vi "GetFrontEndStatus.vi"(8 "error in (no error)":errorcluster) -> (0 "error out":errorcluster, 1 "TestSetDef":T2={"General"={"ID"=0, "Model"="", "Dual Port?"=FALSE, "Options"="", "Options"={"E"=FALSE, "K"=FALSE, "H"=FALSE, "W"=FALSE, "F"=FALSE}, "Cal File"=path ""}, "Receiver"={"Fstart, MHz"=0.0, "Fstop MHz"=0.0, "Fstep MHz"=0.0, "IF, MHz"=0.0}, "RX Band"={"Fstart, MHz"=0.0, "Fstop MHz"=0.0}, "TX 1"={"Fstart, MHz"=0.0, "Fstop MHz"=0.0, "Pmax, dBm"=0.0, "Pstep, dB"=0.0}, "TX 2"={"Fstart, MHz"=0.0, "Fstop MHz"=0.0, "Pmax, dBm"=0.0, "Pstep, dB"=0.0}, "Low-side?"=TRUE}, 2 "Current FE Def":T1, 3 "Saved FE Defs":string[](array[string]), 5 "FE Status Bits":i32)   [LabVIEW 2011]
uses:
  Test Set Definition.ctl
  Front End Definition.ctl
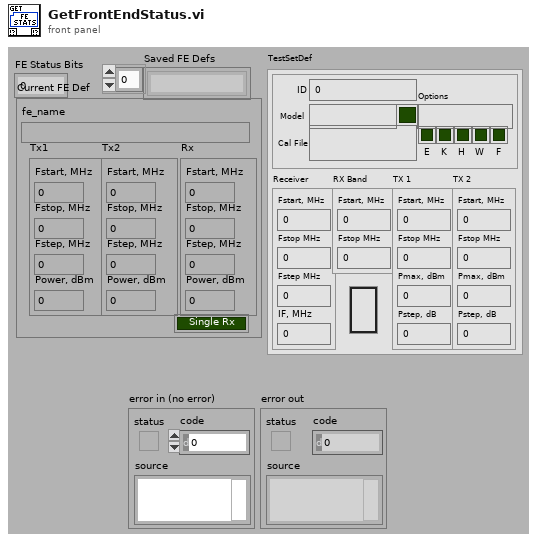
[diagram p1: front panel]
types:
  T1 = typedef "Front End Definition.ctl" = cluster{"fe_name":string, "Tx1":cluster{"Fstart, MHz":dbl, "Fstop, MHz":dbl, "Fstep, MHz":dbl, "Power, dBm":dbl}, "Tx2":cluster{"Fstart, MHz":dbl, "Fstop, MHz":dbl, "Fstep, MHz":dbl, "Power, dBm":dbl}, "Rx":cluster{"Fstart, MHz":dbl, "Fstop, MHz":dbl, "Fstep, MHz":dbl, "Power, dBm":dbl}, "BothSides":bool}
  T2 = typedef "Test Set Definition.ctl" = cluster{"General":cluster{"ID":u32, "Model":string, "Dual Port?":bool, "Options":string, "Options":cluster{"E":bool, "K":bool, "H":bool, "W":bool, "F":bool}, "Cal File":path}, "Receiver":cluster{"Fstart, MHz":dbl, "Fstop MHz":dbl, "Fstep MHz":dbl, "IF, MHz":dbl}, "RX Band":cluster{"Fstart, MHz":dbl, "Fstop MHz":dbl}, "TX 1":cluster{"Fstart, MHz":dbl, "Fstop MHz":dbl, "Pmax, dBm":dbl, "Pstep, dB":dbl}, "TX 2":cluster{"Fstart, MHz":dbl, "Fstop MHz":dbl, "Pmax, dBm":dbl, "Pstep, dB":dbl}, "Low-side?":bool}
  T3 = cluster{"Command":string, "appended array":variant[]}
  T4 = cluster{"Command":string, "appended array":variant[]}[]
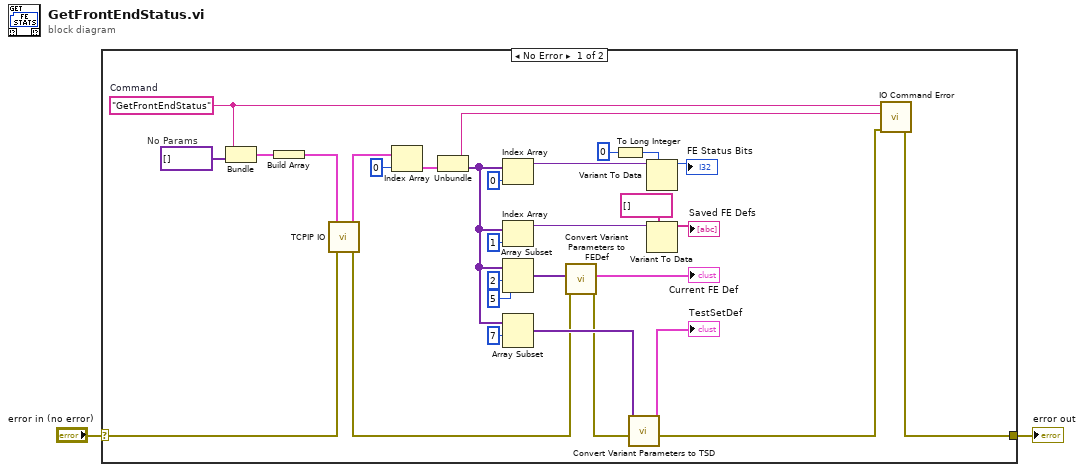
[diagram p0: block diagram]
diagram:
  n1 = case shown="No Error" "error in (no error)" {
    selector: "error in (no error)" -> [w24 w33]
    tunnel: [w30 w33] -> w2
    frame No Error {
      w29 = "GetFrontEndStatus"  # Command
      # "No Params"
      n2 = Bundle("Command"=w29, "appended array"=variant[] []) -> (w32:T3)  [unwired: 1 out]
      n3 = Build Array(w32) -> (w28:T4)
      n4 = call "TCPIP IO.vi"("error in (no error)"=w24, "Commands"=w28) -> ("error out"=w5:errorcluster, "Responses"=w27:cluster{string, variant[]}[])  [unwired: 1 in, 3 out]
      n5 = Index Array(array=w27, index=0) -> (element=w26:cluster{string, variant[]})
      n6 = Unbundle(w26) -> (w25:string, w3:variant[])
      n7 = Index Array(array=w3, index=0) -> (element=w17:variant)
      n8 = Index Array(array=w3, index=1) -> (element=w12:variant)
      n9 = Array Subset(array=w3, index=2, length=5) -> (w7:variant[])
      n10 = Array Subset(array=w3, index=7) -> (w21:variant[])  [unwired: 1 in]
      n11 = call "Convert Variant Parameters to FEDef.vi"("error in"=w5, "Variant Parameter Array"=w7) -> ("error out"=w4:errorcluster, "FE_DEF"=→"Current FE Def":T1)  [unwired: 8 out]
      n12 = To Long Integer(number=0) -> (32bit integer=w18:i32)
      n13 = call "Convert Variant Parameters to TSD.vi"("error in"=w4, "Variant Parameter Array"=w21) -> ("error out"=w22:errorcluster, "TestSetDef"=→"TestSetDef":T2)  [unwired: 8 out]
      n14 = Variant To Data(type=w18, Variant=w17) -> (data=→"FE Status Bits":i32)  [unwired: 1 in, 1 out]
      n15 = Variant To Data(type=string[] [], Variant=w12) -> (data=→"Saved FE Defs":string[])  [unwired: 1 in, 1 out]
      n16 = call "IO Command Error.vi"("error in (no error)"=w22, "Command Returned (\"\")"=w25, "Command Sent (\"\")"=w29) -> ("error out"=w30:errorcluster)  [unwired: 4 out]
    }
    frame Error {
    }
  }
  "error out" <- w2
